vi "SetOvalHeight.vi"(8 "error in (no error)":errorcluster, 10 "Oval Height":i16, 11 "RoundRectangle in":refnum<class "RoundRectangle.lvclass">) -> (0 "error out":errorcluster, 3 "RoundRectangle out":refnum<class "RoundRectangle.lvclass">)   [LabVIEW 2021, in "Picture2D.lvlib" / "RoundRectangle.lvclass"]
uses:
  RoundRectangle.lvclass
  RoundRectangle.lvclass/RoundRectangle.ctl
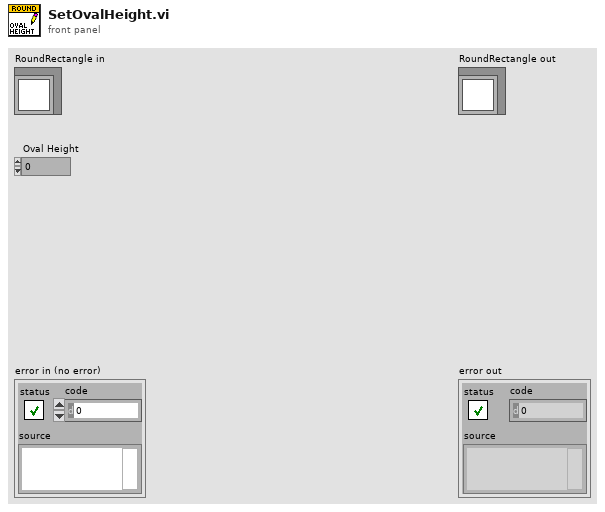
[diagram p1: front panel]
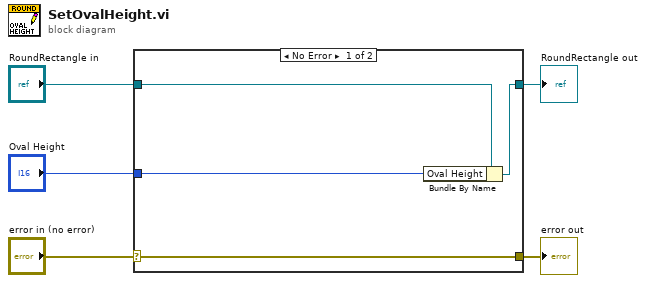
[diagram p0: block diagram]
diagram:
  n1 = case shown="No Error" "error in (no error)" {
    selector: "error in (no error)" -> [w9 w10]
    tunnel: [w9 w10] -> w4
    tunnel: [w7 w11] -> w2
    tunnel: "RoundRectangle in" -> [w8 w11]
    tunnel: "Oval Height" -> [w6 _]
    frame No Error {
      n2 = Bundle By Name(cluster=w8, "Oval Height"=w6) -> (w7:refnum<class "RoundRectangle.lvclass">)
    }
    frame Error {
    }
  }
  "error out" <- w4
  "RoundRectangle out" <- w2
